vi "Pre Launch Init.vi"(11 "Client in":refnum<class "Controller.lvclass">) -> (0 "error out":errorcluster, 3 "Client out":refnum<class "Controller.lvclass">)   [LabVIEW 2023, in "Controller.lvlib" / "Controller.lvclass"]
doc: "(<B>Filename</B>: Actor Framework.lvlib:Actor.lvclass:Pre Launch Init.vi)\n\nDefines behavior that occurs after the Launch Nested Actor method is invoked but before the actor's Actor Core method begins running.\n\nBy default, this method does nothing. A descendant class may override it to define behavior."
uses:
  Controller.lvclass
  Abstraction_Interface_Class/Abstraction_Interface_Class.lvclass
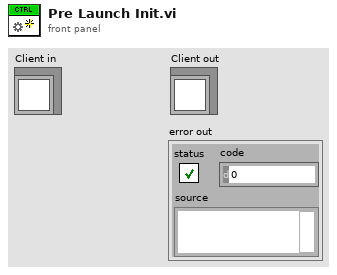
[diagram p1: front panel]
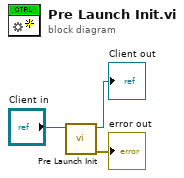
[diagram p0: block diagram]
diagram:
  n1 = call-parent "Pre Launch Init.vi"("Actor in"="Client in") -> ("error out"=→"error out":errorcluster, "Actor out"=→"Client out":refnum<class "Controller.lvclass">)  [unwired: 9 in]
